vi "preprocessing.vi"(10 "RMS":dbl[][](array[numeric])) -> (1 "Vbase":dbl, 2 "Vthresh":dbl, 5 "Incident?":bool)   [LabVIEW 2014]
uses:
  <vilib>/Analysis/NI_AALBase.lvlib
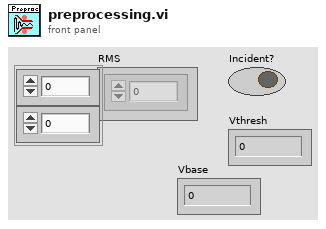
[diagram p1: front panel]
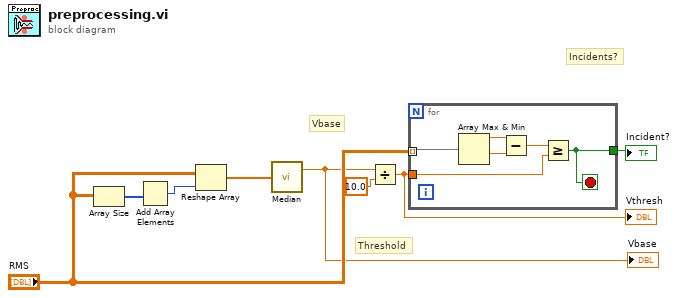
[diagram p0: block diagram]
diagram:
  # "Incidents?"
  # "Threshold"
  # "Vbase"
  n1 = Array Size(array="RMS") -> (size(s)=w8:i32[])
  n2 = Add Array Elements(numeric array=w8) -> (sum=w7:i32)
  n3 = Reshape Array("RMS", w7) -> (w5:dbl[])
  n4 = call <vilib>:"Median.vi"("X"=w5) -> ("median"=w1:dbl)  [unwired: 1 out]
  "Vbase" <- w1
  n5 = Divide(x=w1, y=10.0) -> (x/y=w4:dbl)
  "Vthresh" <- w4
  n6 = for {
    tunnel: "RMS" -> [w14] mode=indexing
    tunnel: [w10] -> w2
    tunnel: w4 -> [w9]
    stop <- w10 stop-if-true
    n7 = Array Max & Min(array=w14) -> (max value=w13:dbl, min value=w12:dbl)  [unwired: 2 out]
    n8 = Subtract(x=w13, y=w12) -> (x-y=w11:dbl)
    n9 = Greater Or Equal?(x=w11, y=w9) -> (x >= y?=w10:bool)
  }
  "Incident?" <- w2
